vi "Fetch Waveform.vi"(6 "Timeout (10000 ms)":i32=10000 min=1, 7 "Trace (0: U1)":i32(ring) items=["U1", "I1", "U2", "I2", "U3", "I3", "U4", "I4", "U5", "I5", "U6", "I6", "Speed", "Torque", "AUX1", "AUX2"], 8 "error in (no error)":errorcluster, 9 "End Point (1600)":i32=1600 min=0 max=1601 step=1, 10 "Start Point (0)":i32 min=0 max=1601 step=1, 11 "VISA resource name":refnum<visa-resource-name>) -> (0 "error out":errorcluster, 2 "Waveform Data":T1(graph), 3 "VISA resource name out":refnum<visa-resource-name>)   [LabVIEW 2021, in "Yokogawa WT1800 Series.lvlib"]
doc: "Returns the waveform the instruments acquired for the specified trace.\n\nThe WT1800 acquires waveforms for the enabled trace concurrently. You must call this VI separately for each enabled channel to obtain the waveforms.\n\nYou can call the Read Waveforms VI instead of using low-level VIs.\n\n<B>Note:</B> \nUse this VI only with other low-level VIs. The high-level VIs automatically incorporate this functionality. This VI does not check the instrument status."
uses:
  <instrlib>/Yokogawa WT1800 Series/Yokogawa WT1800 Series.lvlib
panel:
  # "ms"
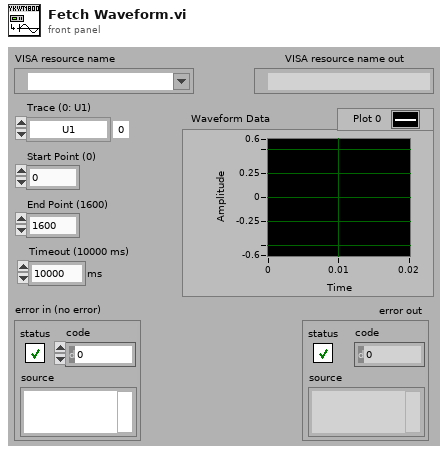
[diagram p1: front panel]
types:
  T1 = cluster{"start":dbl, "Sampling Time":dbl, "Output":dbl[]}
  T2 = cluster{"start":dbl, "Time per Division":dbl, "Output":dbl[]}
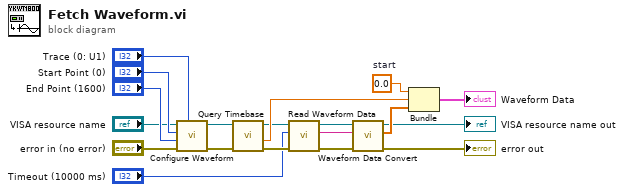
[diagram p0: block diagram]
diagram:
  w18 = 0.0  # start
  n1 = call <instrlib>:"Configure Waveform.vi"("Trace (0: U1)"="Trace (0: U1)", "error in (no error)"="error in (no error)", "End Point (1600)"="End Point (1600)", "Start Point (0)"="Start Point (0)", "VISA resource name"="VISA resource name") -> ("error out"=w4:errorcluster, "VISA resource name out"=w5:refnum<visa-resource-name>)  [unwired: 5 in]
  n2 = call <instrlib>:"Query Timebase.vi"("error in (no error)"=w4, "VISA resource name"=w5) -> ("error out"=w9:errorcluster, "Time per Division"=w17:dbl, "VISA resource name out"=w12:refnum<visa-resource-name>)  [unwired: 7 in]
  n3 = call <instrlib>:"Read Waveform Data.vi"("error in (no error)"=w9, "Timeout (10000 ms)"="Timeout (10000 ms)", "VISA resource name"=w12) -> ("error out"=w10:errorcluster, "Waveform Data"=w19:string, "VISA resource name out"=w11:refnum<visa-resource-name>)  [unwired: 6 in]
  n4 = call <instrlib>:"Waveform Data Convert.vi"("error in (no error)"=w10, "Waveform Data (Empty)"=w19, "VISA resource name"=w11) -> ("error out"=→"error out":errorcluster, "Output"=w16:dbl[], "VISA resource name out"=→"VISA resource name out":refnum<visa-resource-name>)  [unwired: 5 in, 1 out]
  n5 = Bundle("start"=w18, "Time per Division"=w17, "Output"=w16) -> (→"Waveform Data":T2)  [unwired: 1 in]
